vi "Relu.vi"(2 "Z":dbl[][](array[numeric])) -> (0 "Relu(Z)":dbl[][](array[numeric]))   [LabVIEW 2020]
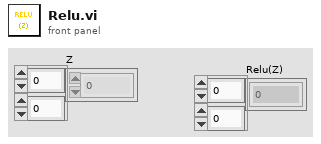
[diagram p1: front panel]
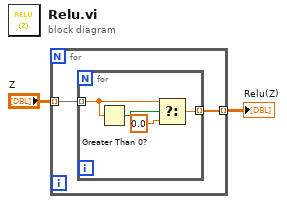
[diagram p0: block diagram]
diagram:
  n1 = for {
    tunnel: "Z" -> [w4] mode=indexing
    tunnel: [w3] -> w1 mode=indexing
    n2 = for {
      tunnel: w4 -> [w7] mode=indexing
      tunnel: [w5] -> w3 mode=indexing
      n3 = Greater Than 0?(x=w7) -> (x > 0?=w8:bool)
      n4 = Select(t=w7, s=w8, f=0.0) -> (s? t:f=w5:dbl)
    }
  }
  "Relu(Z)" <- w1
